vi "rethinkdb_json_stack.vi"(7 "action":enum8{"push", "pop"}(ring), 8 "error in (no error)":errorcluster, 9 "value":variant, 10 "name":string, 11 "stack in":T1(array[cluster])) -> (0 "error out":errorcluster, 3 "stack out":T1(array[cluster]))   [LabVIEW 2017]
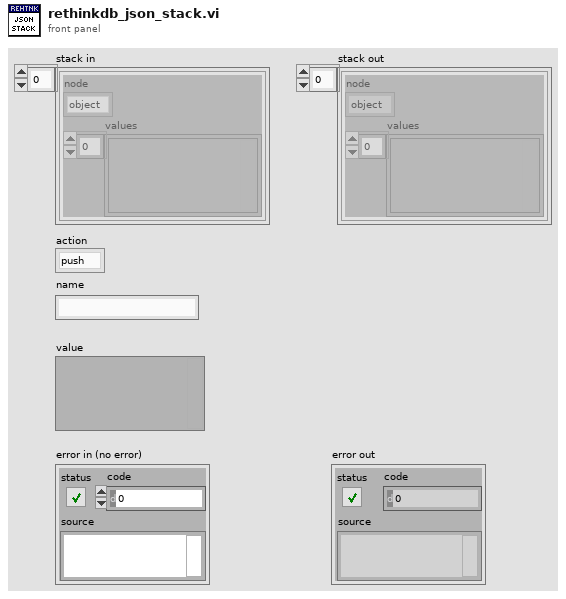
[diagram p1: front panel]
types:
  T1 = cluster{"node":enum8{"object", "array"}, "values":variant[]}[]
  T2 = cluster{"node":enum8{"object", "array"}, "values":variant[]}
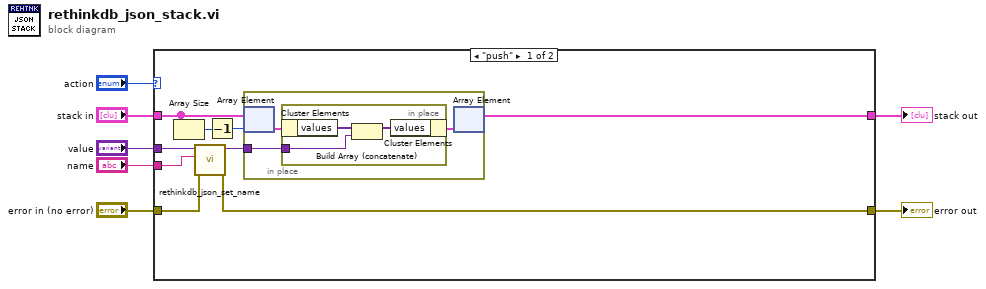
[diagram p0: block diagram]
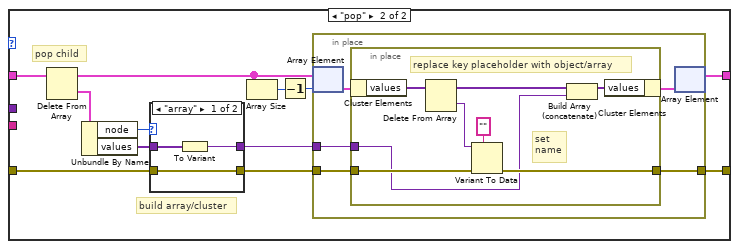
[diagram p2: hidden frame]
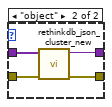
[diagram p3: hidden frame]
diagram:
  n1 = case shown="\"push\"" "action" {
    tunnel: [w16 w34] -> w7
    tunnel: "value" -> [w10 _]
    tunnel: "stack in" -> [w14 w31]
    tunnel: "error in (no error)" -> [w12 w27]
    tunnel: [w11 w28] -> w2
    tunnel: "name" -> [w8 _]
    frame "push" {
      n2 = Array Size(array=w14) -> (size(s)=w13:i32)
      n3 = call "rethinkdb_json_set_name.vi"("error in (no error)"=w12, "name"=w8, "variant in"=w10) -> ("error out"=w11:errorcluster, "variant out"=w9:variant)  [unwired: 7 in]
      n4 = Decrement(x=w13) -> (x-1=w15:i32)
      n5 = in-place {
        in-place-border: w9 -> [w18]
        n6 = in-place-array #1(w14, w15) -> (w19:T2)
        n7 = in-place {
          in-place-border: w18 -> [w20]
          n8 = in-place-cluster #2(w19) -> ("values"=w22:variant[])
          n9 = Build Array (concatenate)(w22, w20) -> (w21:variant[])
          n10 = in-place-cluster #2("values"=w21) -> (w17:T2)
        }
        n11 = in-place-array #1(w17) -> (w16:T1)  [unwired: 1 out]
      }
    }
    frame "pop" {
      # "build array/cluster"
      # "pop child"
      n12 = Delete From Array(array=w31) -> (deleted portion=w29:T2, array with subset deleted=w30:T1)  [unwired: 2 in]
      n13 = Unbundle By Name(w29) -> ("node"=w24:enum8{"object", "array"}, "values"=w25:variant[])
      n14 = case shown="\"array\"" w24 {
        tunnel: w27 -> [w36 w41]
        tunnel: [w36 w40] -> w26
        tunnel: w25 -> [w37 w39]
        tunnel: [w35 w38] -> w23
        frame "array" {
          n15 = To Variant(anything=w37) -> (Variant=w35:variant)
        }
        frame "object" {
          n16 = call "rethinkdb_json_cluster_new.vi"("error in (no error)"=w41, "elements"=w39) -> ("error out"=w40:errorcluster, "cluster"=w38:variant)  [unwired: 8 in]
        }
      }
      n17 = Array Size(array=w30) -> (size(s)=w32:i32)
      n18 = Decrement(x=w32) -> (x-1=w33:i32)
      n19 = in-place {
        in-place-border: w26 -> [w44]
        in-place-border: [w43] -> w28
        in-place-border: w23 -> [w42]
        n20 = in-place-array #3(w30, w33) -> (w46:T2)
        n21 = in-place {
          in-place-border: w44 -> [w49]
          in-place-border: [w48] -> w43
          in-place-border: w42 -> [w47]
          # "replace key placeholder with object/array"
          # "set\nname"
          n22 = in-place-cluster #4(w46) -> ("values"=w53:variant[])
          n23 = Delete From Array(array=w53) -> (deleted portion=w51:variant, array with subset deleted=w52:variant[])  [unwired: 2 in]
          n24 = Variant To Data(error in=w49, type="", Variant=w51) -> (error out=w48:errorcluster)  [unwired: 1 out]
          n25 = Build Array (concatenate)(w52, w47) -> (w54:variant[])
          n26 = in-place-cluster #4("values"=w54) -> (w45:T2)
        }
        n27 = in-place-array #3(w45) -> (w34:T1)  [unwired: 1 out]
      }
    }
  }
  "stack out" <- w7
  "error out" <- w2
